vi "RandomPick.vi"(11 "DataIn":T1) -> (3 "DataOut":dbl[](array[numeric]))   [LabVIEW 2018, in "DataDisplay.lvlib"]
uses:
  DataDisplay.lvlib
  TypeDefine/DD_DataStream.ctl
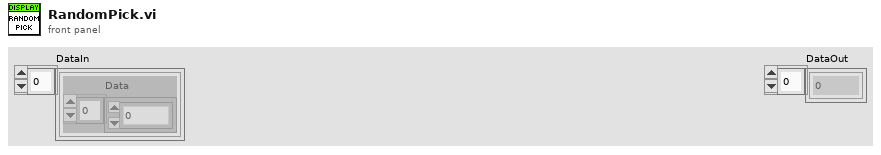
[diagram p1: front panel]
types:
  T1 = typedef "DataDisplay.lvlib/DD_DataStream.ctl" = cluster{"Data":dbl[]}[]
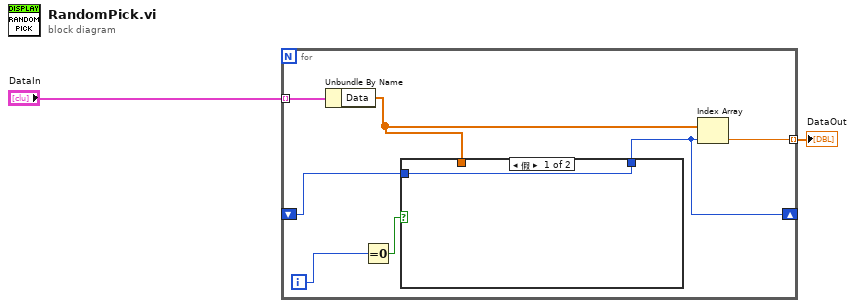
[diagram p0: block diagram]
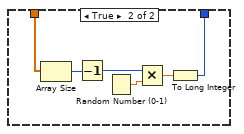
[diagram p2: hidden frame]
diagram:
  n1 = for {
    tunnel: "DataIn" -> [w9] mode=indexing
    tunnel: [w8] -> w1 mode=indexing
    shift-right: [w4] -> _
    shift-left: _ -> [w3]
    i -> [w7]
    n2 = Unbundle By Name(w9) -> ("Data"=w5:dbl[])
    n3 = Equal To 0?(x=w7) -> (x = 0?=w6:bool)
    n4 = case shown="假" w6 {
      tunnel: w5 -> [_ w12]
      tunnel: [w10 w11] -> w4
      tunnel: w3 -> [w10 _]
      frame False {
      }
      frame True {
        n5 = Array Size(array=w12) -> (size(s)=w16:i32)
        n6 = Decrement(x=w16) -> (x-1=w13:i32)
        n7 = Random Number (0-1)() -> (number: 0 to 1=w15:dbl)
        n8 = Multiply(x=w13, y=w15) -> (x*y=w14:dbl)
        n9 = To Long Integer(number=w14) -> (32bit integer=w11:i32)
      }
    }
    n10 = Index Array(array=w5, index=w4) -> (element=w8:dbl)
  }
  "DataOut" <- w1
